vi "Parameter Info.vi"(7 "Board parameter? (F)":bool, 8 "error in (no error)":errorcluster, 9 "Parameter name":string, 10 "Channel":i8, 11 "BoardHandle":T2) -> (0 "error out":errorcluster, 2 "Parameter descriptor":T1, 3 "BoardHandle out":T2)   [LabVIEW 2020, in "CAEN PSM.lvlib"]
doc: "This function returns information of a parameter indicated in the input (both of board and channel)."
uses:
  CAEN PSM.lvlib
  BoardHandle.ctl
  DeviceFamily.ctl
  <vilib>/regexp/Match Regular Expression.xnode
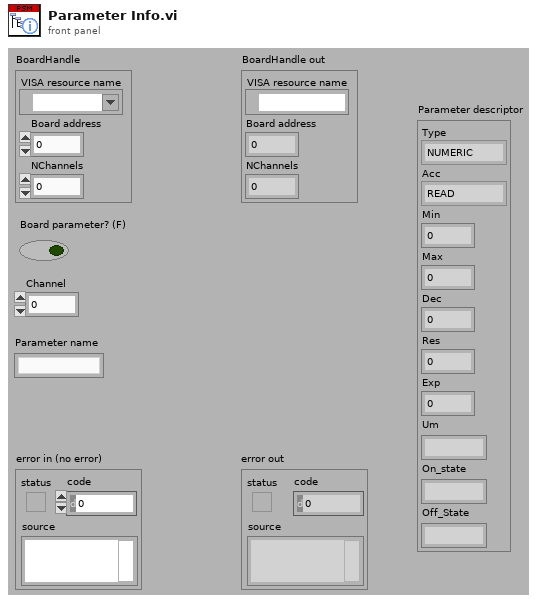
[diagram p1: front panel]
types:
  T1 = cluster{"Type":enum16{"NUMERIC", "ONOFF", "CHSTATUS", "BDSTATUS", "BINARY", "STRING", "ENUM"}, "Acc":enum16{"READ", "WRITE", "READ_WRITE"}, "Min":u32, "Max":u32, "Dec":u32, "Res":u32, "Exp":i32, "Um":string, "On_state":string, "Off_State":string}
  T2 = typedef "CAEN PSM.lvlib/BoardHandle.ctl" = cluster{"VISA resource name":refnum<visa-resource-name>, "Board address":i8, "NChannels":u8}
  T3 = typedef "CAEN PSM.lvlib/DeviceFamily.ctl" = enum8{"NIM / DESKTOP HV", "DT55XXE HV", "SMART HV"}
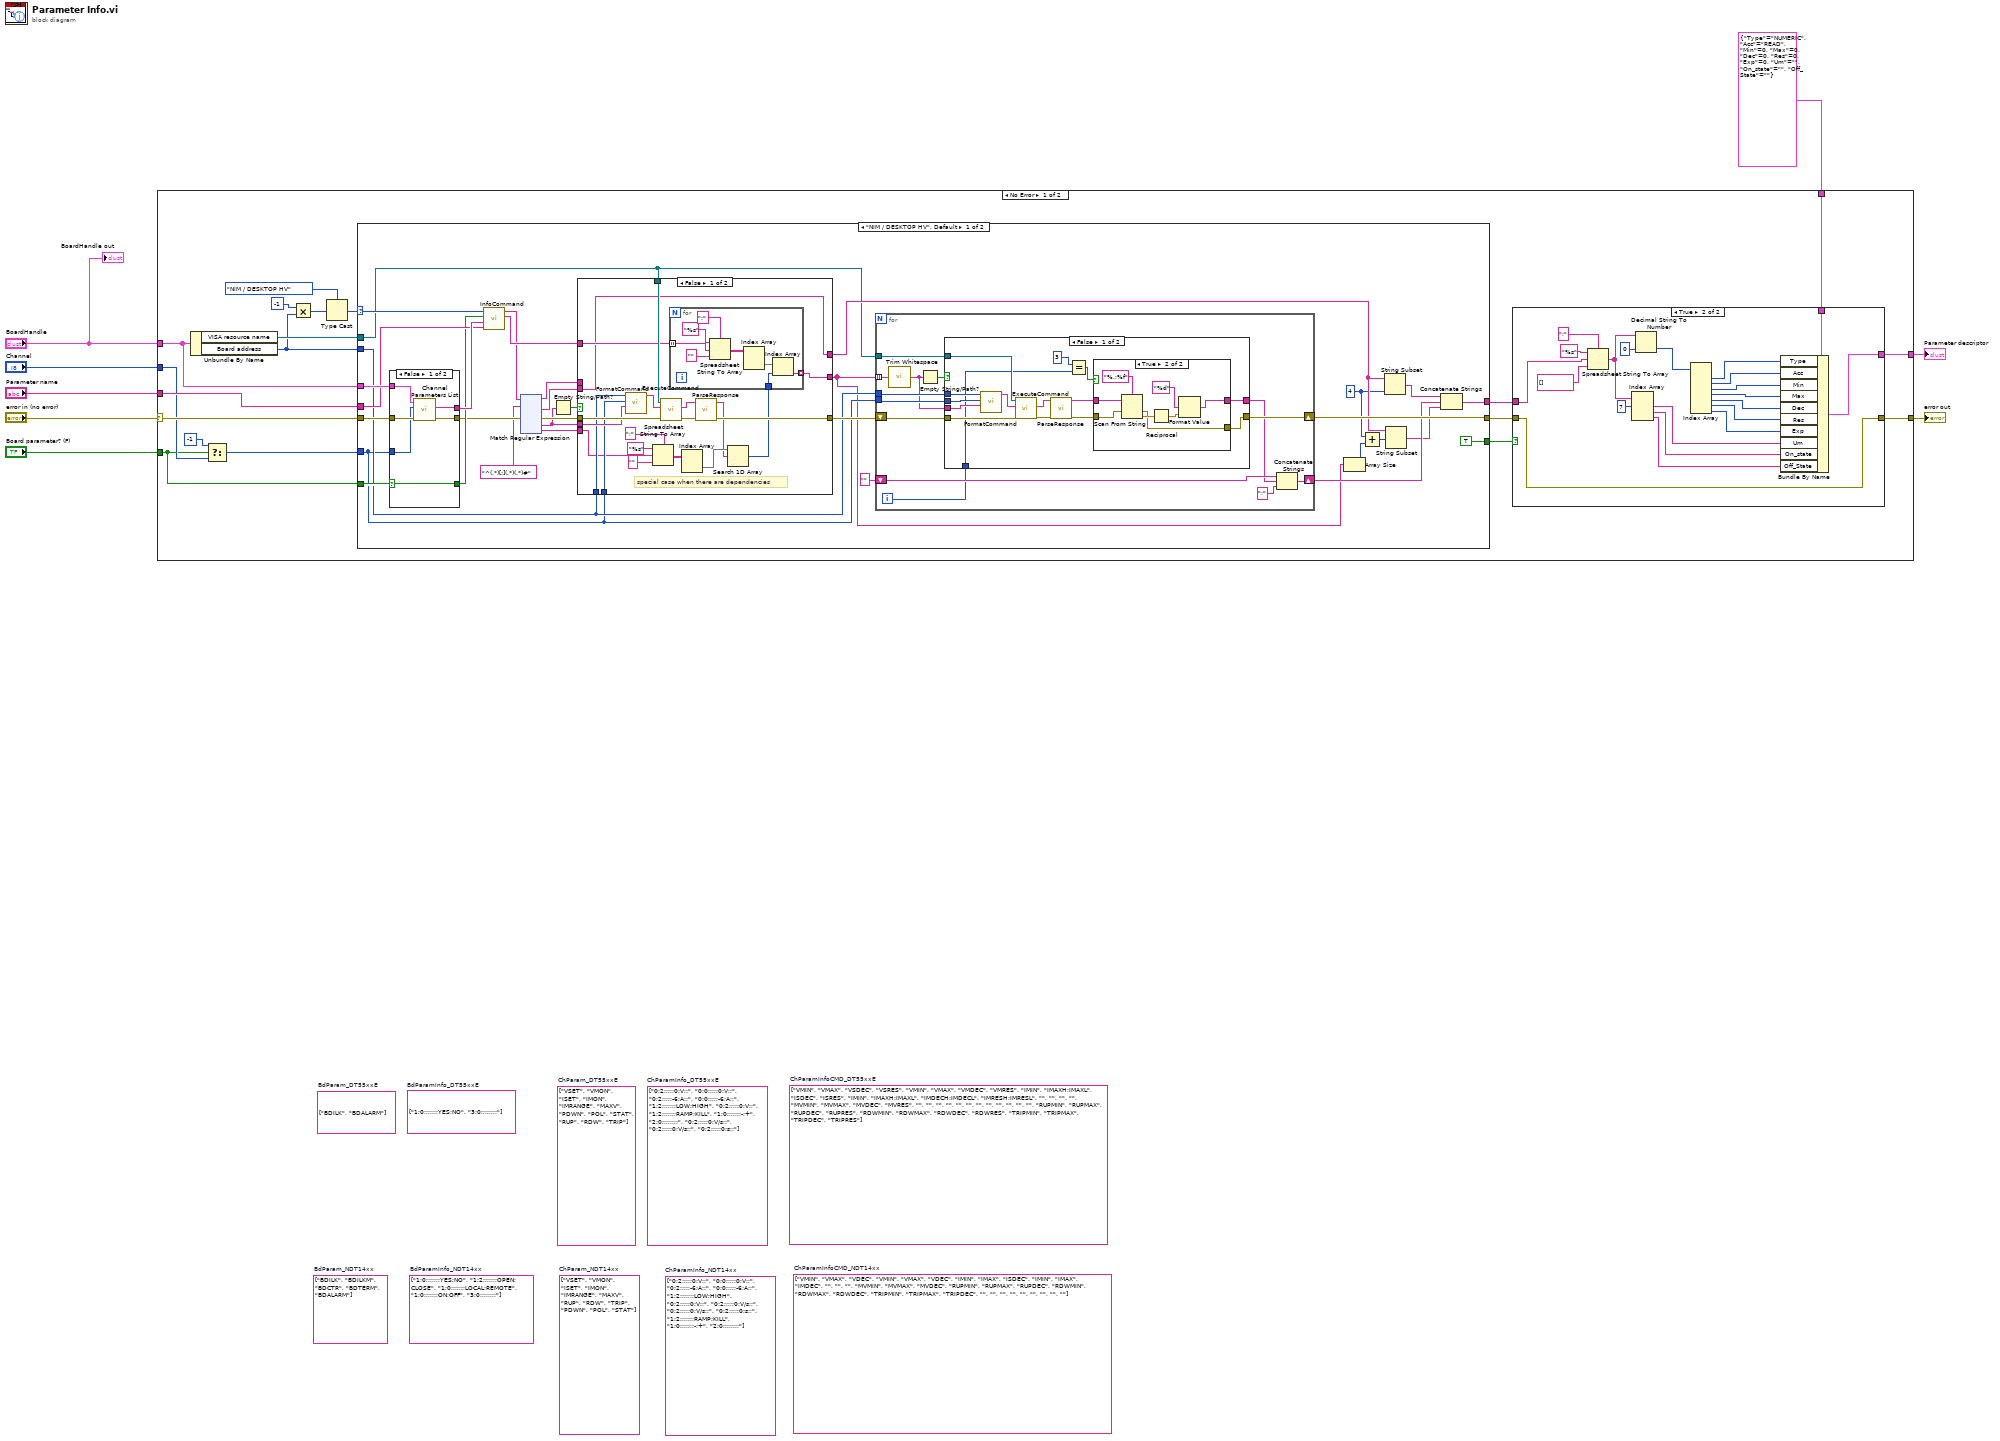
[diagram p0: block diagram]
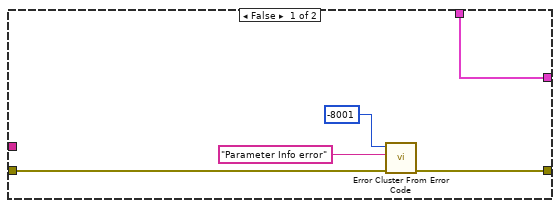
[diagram p2: hidden frame]
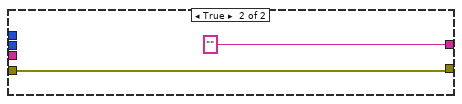
[diagram p5: hidden frame]
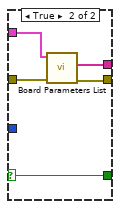
[diagram p6: hidden frame]
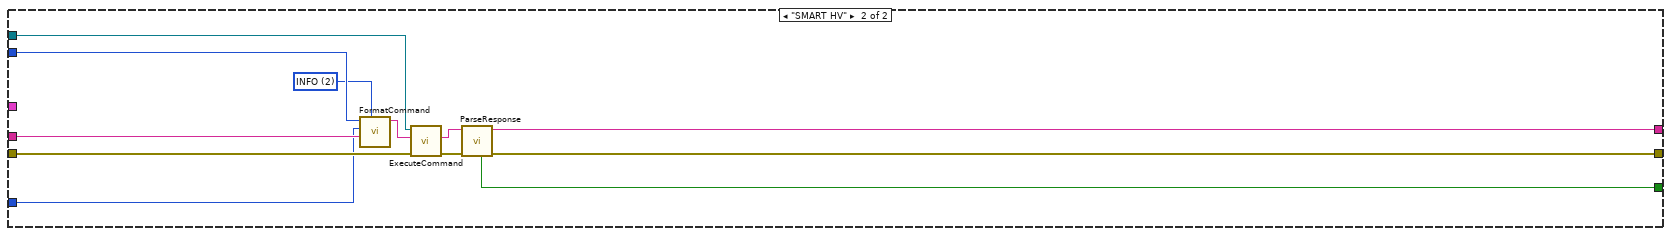
[diagram p7: hidden frame]
diagram:
  (unwired) string[][] [["VMIN", "VMAX", "VDEC"], ["VMIN", "VMAX", "VDEC"], ["IMIN", "IMAX", "ISDEC"], ["IMIN", "IMAX", "IMDEC"], ["", "", ""], ["MVMIN", "MVMAX", "MVDEC"], ["RUPMIN", "RUPMAX", "RUPDEC"], ["RDWMIN", "RDWMAX", "RDWDEC"], ["TRIPMIN", "TRIPMAX", "TRIPDEC"], ["", "", ""], ["", "", ""], ["", "", ""]]  # ChParamInfoCMD_NDT14xx
  (unwired) string[] ["0;2;;;;;0;V;;", "0;0;;;;;0;V;;", "0;2;;;;;-6;A;;", "0;0;;;;;-6;A;;", "1;2;;;;;;;LOW;HIGH", "0;2;;;;;0;V;;", "0;2;;;;;0;V/s;;", "0;2;;;;;0;V/s;;", "0;2;;;;;0;s;;", "1;2;;;;;;;RAMP;KILL", "1;0;;;;;;;-;+", "2;0;;;;;;;;"]  # ChParamInfo_NDT14xx
  (unwired) string[] ["1;0;;;;;;;YES;NO", "1;2;;;;;;;OPEN; CLOSE", "1;0;;;;;;;LOCAL;REMOTE", "1;0;;;;;;;ON;OFF", "3;0;;;;;;;;"]  # BdParamInfo_NDT14xx
  (unwired) string[] ["VSET", "VMON", "ISET", "IMON", "IMRANGE", "MAXV", "RUP", "RDW", "TRIP", "PDWN", "POL", "STAT"]  # ChParam_NDT14xx
  (unwired) string[] ["BDILK", "BDILKM", "BDCTR", "BDTERM", "BDALARM"]  # BdParam_NDT14xx
  (unwired) string[][] [["VMIN", "VMAX", "VSDEC", "VSRES"], ["VMIN", "VMAX", "VMDEC", "VMRES"], ["IMIN", "IMAXH;IMAXL", "ISDEC", "ISRES"], ["IMIN", "IMAXH;IMAXL", "IMDECH;IMDECL", "IMRESH;IMRESL"], ["", "", "", ""], ["MVMIN", "MVMAX", "MVDEC", "MVRES"], ["", "", "", ""], ["", "", "", ""], ["", "", "", ""], ["RUPMIN", "RUPMAX", "RUPDEC", "RUPRES"], ["RDWMIN", "RDWMAX", "RDWDEC", "RDWRES"], ["TRIPMIN", "TRIPMAX", "TRIPDEC", "TRIPRES"]]  # ChParamInfoCMD_DT55xxE
  (unwired) string[] ["0;2;;;;;0;V;;", "0;0;;;;;0;V;;", "0;2;;;;;-6;A;;", "0;0;;;;;-6;A;;", "1;2;;;;;;;LOW;HIGH", "0;2;;;;;0;V;;", "1;2;;;;;;;RAMP;KILL", "1;0;;;;;;;-;+", "2;0;;;;;;;;", "0;2;;;;;0;V/s;;", "0;2;;;;;0;V/s;;", "0;2;;;;;0;s;;"]  # ChParamInfo_DT55xxE
  (unwired) string[] ["1;0;;;;;;;YES;NO", "3;0;;;;;;;;"]  # BdParamInfo_DT55xxE
  (unwired) string[] ["VSET", "VMON", "ISET", "IMON", "IMRANGE", "MAXV", "PDWN", "POL", "STAT", "RUP", "RDW", "TRIP"]  # ChParam_DT55xxE
  (unwired) string[] ["BDILK", "BDALARM"]  # BdParam_DT55xxE
  n1 = case shown="No Error" "error in (no error)" {
    selector: "error in (no error)" -> [w27 w299]
    tunnel: [w14 w299] -> w7
    tunnel: "BoardHandle" -> [w15 _]
    tunnel: "Channel" -> [w23 _]
    tunnel: "Parameter name" -> [w25 _]
    tunnel: "Board parameter? (F)" -> [w16 _]
    tunnel: [w12 w298] -> w1
    tunnel: T1 {"Type"=enum."NUMERIC", "Acc"=enum."READ", "Min"=0, "Max"=0, "Dec"=0, "Res"=0, "Exp"=0, "Um"="", "On_state"="", "Off_State"=""} ("Parameter descriptor") -> [w11 w298]
    frame No Error {
      n2 = Unbundle By Name(w15) -> ("VISA resource name"=w26:refnum<visa-resource-name>, "Board address"=w18:i8)
      n3 = Select(t=i8 -1, s=w16, f=w23) -> (s? t:f=w22:i8)
      n4 = Multiply(x=i8 -1, y=w18) -> (x*y=w20:i8)
      n5 = Type Cast(type=DeviceFamily."NIM / DESKTOP HV" ("Device Family"), x=w20) -> (*(type *) &x=w17:T3)
      n6 = case shown="\"NIM / DESKTOP HV\", Default" w17 {
        selector: w17 -> [w84 _]
        tunnel: w27 -> [w86 w294]
        tunnel: w26 -> [w62 w293]
        tunnel: w18 -> [w59 w292]
        tunnel: w25 -> [w81 w290]
        tunnel: w22 -> [w58 w289]
        tunnel: [w79 w288] -> w13
        tunnel: w16 -> [w83 _]
        tunnel: w15 -> [w85 _]
        tunnel: [w78 w287] -> w10
        tunnel: [TRUE ("OK") w286] -> w9
        frame "NIM / DESKTOP HV", Default {
          w56 = 4 ("length (rest)")
          n7 = case shown="False" w83 {
            selector: w83 -> [w275 w281]
            tunnel: w86 -> [w280 w285]
            tunnel: w85 -> [w279 w284]
            tunnel: w58 -> [w278 _]
            tunnel: [w277 w283] -> w82
            tunnel: [w276 w282] -> w70
            tunnel: [w275 w281] -> w73
            frame False {
              n8 = call "Channel Parameters List.vi"("error in (no error)"=w280, "Channel (0)"=w278, "BoardHandle"=w279) -> ("error out"=w276:errorcluster, "Parameters list"=w277:string[])  [unwired: 5 in, 2 out]
            }
            frame True {
              n9 = call "Board Parameters List.vi"("error in (no error)"=w285, "BoardHandle"=w284) -> ("error out"=w282:errorcluster, "Parameters list"=w283:string[])  [unwired: 6 in, 2 out]
            }
          }
          n10 = call "InfoCommand.vi"("PAR"=w81, "Parameters list"=w82, "Board parameter? (F)"=w73, "Device Family"=w84) -> ("info_commands"=w71:string[], "info_response"=w66:string)  [unwired: 6 in]
          n11 = xnode "Match Regular Expression"("input string"=w66, "regular expression"="^(.*)[:](.*)(.*)#", "error in"=w70) -> ("before match"=w64:string, "after match"=w60:string, "error out"=w69:errorcluster, "submatch 1"=w63:string, "submatch 2"=w61:string)  [unwired: 3 in, 2 out]
          n12 = Empty String/Path?(string/path=w63) -> (empty?=w67:bool)
          n13 = case shown="False" w67 {
            tunnel: w69 -> [w223 w234]
            tunnel: [w215 w234] -> w72
            tunnel: w71 -> [w207 w233]
            tunnel: [w205 w233] -> w54
            tunnel: [w204 w232] -> w65
            tunnel: w64 -> [_ w232]
            tunnel: w63 -> [w221 _]
            tunnel: w59 -> [w220 _]
            tunnel: w58 -> [w219 _]
            tunnel: w62 -> [w218 _]
            tunnel: w61 -> [w210 _]
            tunnel: w60 -> [w204 _]
            frame False {
              # "special case when there are dependencies"
              n14 = call "FormatCommand.vi"("PAR"=w221, "CH"=w219, "BD (0)"=w220) -> ("cmd"=w217:string)  [unwired: 8 in]
              n15 = Spreadsheet String To Array(delimiter (Tab)=";", format string="%s", spreadsheet string=w210, array type (2D Dbl)="") -> (array=w214:string[][])
              n16 = call "ExecuteCommand.vi"("error in (no error)"=w223, "Command"=w217, "VISA resource name"=w218) -> ("error out"=w222:errorcluster, "Response"=w216:string)  [unwired: 6 in, 1 out]
              n17 = Index Array(array=w214) -> (element=w209:string[])  [unwired: 2 in]
              n18 = call "ParseResponse.vi"("error in (no error)"=w222, "Response"=w216) -> ("error out"=w215:errorcluster, "val"=w208:string)  [unwired: 6 in, 2 out]
              n19 = Search 1D Array(1D array=w209, element=w208) -> (index of element=w206:i32)  [unwired: 1 in]
              n20 = for {
                tunnel: w207 -> [w231] mode=indexing
                tunnel: w206 -> [w225]
                tunnel: [w224] -> w205 mode=indexing
                n21 = Spreadsheet String To Array(delimiter (Tab)=";", format string="%s", spreadsheet string=w231, array type (2D Dbl)="") -> (array=w227:string[][])
                n22 = Index Array(array=w227) -> (element=w226:string[])  [unwired: 2 in]
                n23 = Index Array(array=w226, index=w225) -> (element=w224:string)
              }
            }
            frame True {
              # "standard case"
            }
          }
          n24 = for {
            tunnel: w54 -> [w247] mode=indexing
            tunnel: w59 -> [w244]
            tunnel: w58 -> [w243]
            shift-right: [w241] -> w79
            shift-left: w72 -> [w245]
            shift-right: [w240] -> w76
            shift-left: "" -> [w239]
            tunnel: w62 -> [w236]
            i -> [w235]
            n25 = call <vilib>:"Trim Whitespace.vi"("string"=w247) -> ("trimmed string"=w242:string)  [unwired: 1 in]
            n26 = Empty String/Path?(string/path=w242) -> (empty?=w246:bool)
            n27 = case shown="False" w246 {
              tunnel: w245 -> [w259 w273]
              tunnel: w244 -> [w258 _]
              tunnel: w243 -> [w257 _]
              tunnel: w242 -> [w256 _]
              tunnel: [w251 "" ("val")] -> w238
              tunnel: [w249 w273] -> w241
              tunnel: w236 -> [w255 _]
              tunnel: w235 -> [w253 _]
              frame False {
                n28 = call "FormatCommand.vi"("PAR"=w256, "CH"=w257, "BD (0)"=w258) -> ("cmd"=w262:string)  [unwired: 8 in]
                n29 = call "ExecuteCommand.vi"("error in (no error)"=w259, "Command"=w262, "VISA resource name"=w255) -> ("error out"=w261:errorcluster, "Response"=w260:string)  [unwired: 6 in, 1 out]
                n30 = call "ParseResponse.vi"("error in (no error)"=w261, "Response"=w260) -> ("error out"=w250:errorcluster, "val"=w252:string)  [unwired: 6 in, 2 out]
                n31 = Equal?(x=3 ("y"), y=w253) -> (x = y?=w248:bool)
                n32 = case shown="True" w248 {
                  tunnel: w252 -> [w264 w265]
                  tunnel: [w264 w271] -> w251
                  tunnel: w250 -> [w263 w267]
                  tunnel: [w263 w266] -> w249
                  frame False {
                  }
                  frame True {
                    n33 = Scan From String(format string="%.;%f", input string=w265, error in=w267) -> (error out=w266:errorcluster, output 1=w268:dbl)  [unwired: 2 in, 2 out]
                    n34 = Reciprocal(x=w268) -> (1/x=w272:dbl)
                    n35 = Format Value(format string="%d", value (0)=w272) -> (output string=w271:string)  [unwired: 1 in]
                  }
                }
              }
              frame True {
              }
            }
            n36 = Concatenate Strings(w239, w238, ";" ("string")) -> (w240:string)
          }
          n37 = Array Size(array=w54) -> (size(s)=w55:i32)
          n38 = Add(x=w56, y=w55) -> (x+y=w57:i32)
          n39 = String Subset(string=w65, length (rest)=w56) -> (substring=w77:string)  [unwired: 1 in]
          n40 = String Subset(string=w65, offset (0)=w57) -> (substring=w75:string)  [unwired: 1 in]
          n41 = Concatenate Strings(w77, w76, w75) -> (w78:string)
        }
        frame "SMART HV" {
          w291 = u8 2 items=["MON", "SET", "INFO"] ("CMD (MON)")
          n42 = call "FormatCommand.vi"("CMD (MON)"=w291, "PAR"=w290, "CH"=w289, "BD (0)"=w292) -> ("cmd"=w297:string)  [unwired: 7 in]
          n43 = call "ExecuteCommand.vi"("error in (no error)"=w294, "Command"=w297, "VISA resource name"=w293) -> ("error out"=w296:errorcluster, "Response"=w295:string)  [unwired: 6 in, 1 out]
          n44 = call "ParseResponse.vi"("error in (no error)"=w296, "Response"=w295) -> ("error out"=w288:errorcluster, "val"=w287:string, "OK"=w286:bool)  [unwired: 6 in, 1 out]
        }
      }
      n45 = case shown="True" w9 {
        tunnel: w10 -> [_ w51]
        tunnel: w13 -> [w30 w47]
        tunnel: [w31 w47] -> w14
        tunnel: [w32 w48] -> w12
        tunnel: w11 -> [w32 w49]
        frame False {
          n46 = call <vilib>:"Error Cluster From Error Code.vi"("error in (no error)"=w30, "error message (\"\")"="Parameter Info error" ("error message (\"\")"), "error code (0)"=-8001) -> ("error out"=w31:errorcluster)  [unwired: 6 in]
        }
        frame True {
          n47 = Spreadsheet String To Array(delimiter (Tab)=";", format string="%s", spreadsheet string=w51, array type (2D Dbl)=string[] []) -> (array=w43:string[])
          n48 = Index Array(array=w43, index #1=7 ("index")) -> (element #1=w44:string, element #2=w45:string, element #3=w46:string)  [unwired: 2 in]
          n49 = Decimal String To Number(string=w43, default (0L)=0 ("default (0 I32)")) -> (number=w41:i32[])  [unwired: 1 in, 1 out]
          n50 = Index Array(array=w41) -> (element #1=w40:i32, element #2=w39:i32, element #3=w38:i32, element #4=w37:i32, element #5=w36:i32, element #6=w35:i32, element #7=w34:i32)  [unwired: 7 in]
          n51 = Bundle By Name(cluster=w49, "Type"=w40, "Acc"=w39, "Min"=w38, "Max"=w37, "Dec"=w36, "Res"=w35, "Exp"=w34, "Um"=w44, "On_state"=w45, "Off_State"=w46) -> (w48:T1)
        }
      }
    }
    frame Error {
    }
  }
  "error out" <- w7
  "Parameter descriptor" <- w1
  "BoardHandle out" <- "BoardHandle"
